vi "ProcessJSONRun.vi"(8 "error in (no error)":errorcluster, 11 "JSON Array":string) -> (0 "error out":errorcluster, 2 "JSON Response String":string, 3 "JSON Error string":string)   [LabVIEW 2013]
uses:
  <vilib>/regexp/Match Regular Expression.xnode
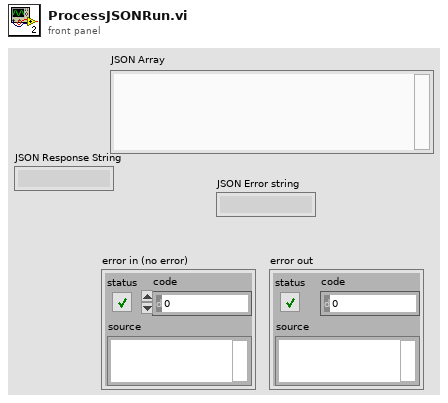
[diagram p1: front panel]
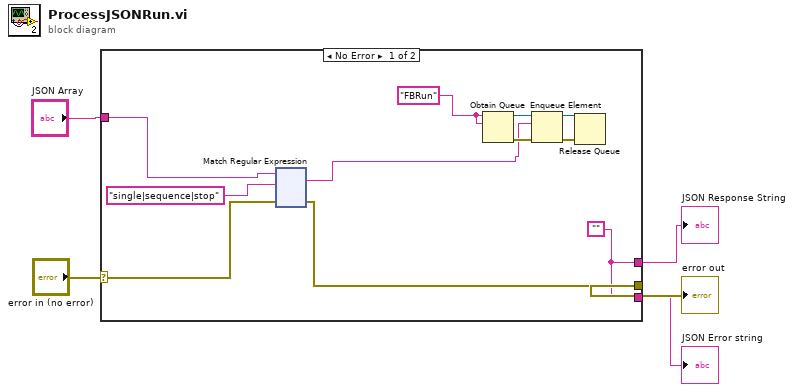
[diagram p0: block diagram]
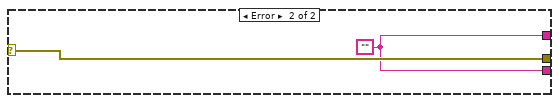
[diagram p2: hidden frame]
diagram:
  n1 = case shown="No Error" "error in (no error)" {
    selector: "error in (no error)" -> [w7 w132]
    tunnel: "JSON Array" -> [w10 _]
    tunnel: [w6 w132] -> w5
    tunnel: [w16 w131] -> w3
    tunnel: [w16 w131] -> w2
    frame No Error {
      w11 = "FBRun" ("name (unnamed)")
      w16 = ""
      n2 = xnode "Match Regular Expression"("input string"=w10, "regular expression"="single|sequence|stop", "error in"=w7) -> ("whole match"=w8:string, "error out"=w6:errorcluster)  [unwired: 3 in, 3 out]
      n3 = Obtain Queue(name (unnamed)=w11, element data type=w11) -> (queue out=w15:refnum<queue>, error out=w14:errorcluster)  [unwired: 3 in, 1 out]
      n4 = Enqueue Element(queue=w15, element=w8, error in (no error)=w14) -> (queue out=w13:refnum<queue>, error out=w12:errorcluster)  [unwired: 1 in, 1 out]
      n5 = Release Queue(queue=w13, error in (no error)=w12) -> ()  [unwired: 1 in, 3 out]
    }
    frame Error {
      w131 = ""
    }
  }
  "error out" <- w5
  "JSON Error string" <- w3
  "JSON Response String" <- w2
